vi "ContFindIterationStart.vi"(11 "ItemNames":string[][](array[string])) -> (3 "Array":i32[][](array[numeric]))   [LabVIEW 2018, in "Config.lvlib"]
uses:
  Config/Config.lvlib
  <vilib>/regexp/Match Regular Expression.xnode
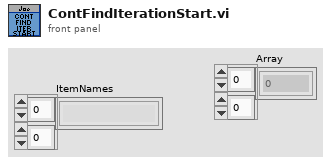
[diagram p1: front panel]
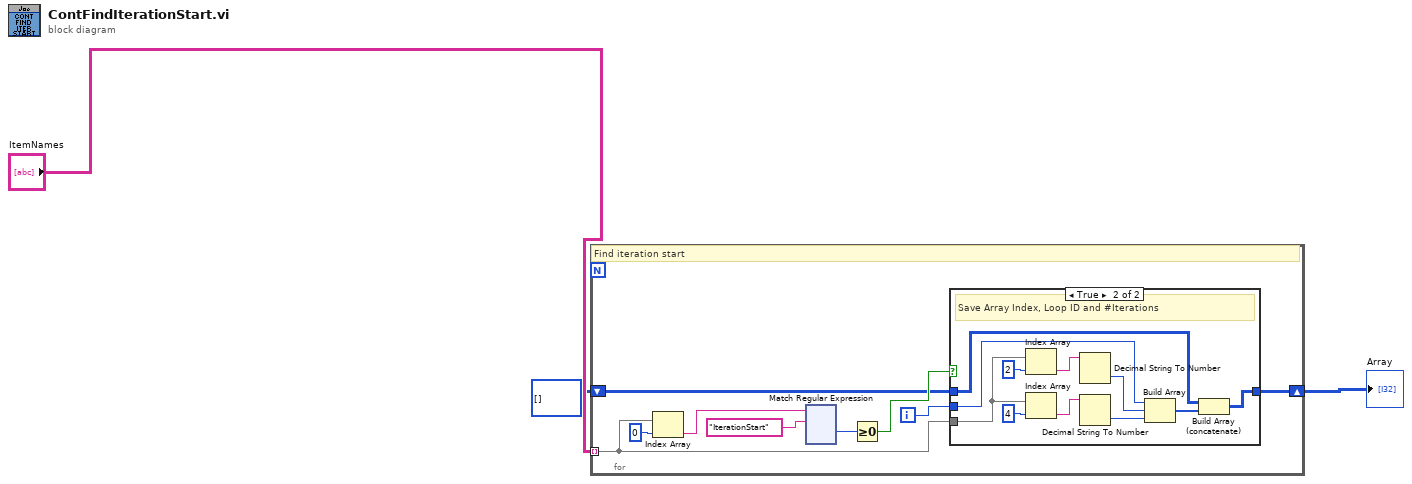
[diagram p0: block diagram]
diagram:
  n1 = for {
    shift-right: [w9] -> w2
    shift-left: i32[][] [] -> [w8]
    tunnel: "ItemNames" -> [w5] mode=indexing
    i -> [w4]
    # "Find iteration start"
    n2 = Index Array(array=w5, index=0 ("disabled index (col)")) -> (element=w7:string)
    n3 = xnode "Match Regular Expression"("input string"=w7, "regular expression"="IterationStart" ("element")) -> ("offset past match"=w11:i32)  [unwired: 4 in, 4 out]
    n4 = Greater Or Equal To 0?(x=w11) -> (x >= 0?=w10:bool)
    n5 = case shown="True" w10 {
      tunnel: [w13 w24] -> w9
      tunnel: w8 -> [w13 w23]
      tunnel: w5 -> [_ w16]
      tunnel: w4 -> [_ w22]
      frame False {
      }
      frame True {
        # "Save Array Index, Loop ID and #Iterations"
        n6 = Index Array(array=w16, index=2 ("disabled index (col)")) -> (element=w19:string)
        n7 = Index Array(array=w16, index=4 ("disabled index (col)")) -> (element=w17:string)
        n8 = Decimal String To Number(string=w19) -> (number=w15:i32)  [unwired: 2 in, 1 out]
        n9 = Decimal String To Number(string=w17) -> (number=w14:i32)  [unwired: 2 in, 1 out]
        n10 = Build Array(w22, w15, w14) -> (w21:i32[])
        n11 = Build Array (concatenate)(w23, w21) -> (w24:i32[][])
      }
    }
  }
  "Array" <- w2
